vi "Reset Error Status.vi"(8 "error in (no error)":errorcluster, 11 "navX Error Status in":refnum<class "navX Error Status.lvclass">) -> (0 "error out":errorcluster, 3 "navX Error Status out":refnum<class "navX Error Status.lvclass">)   [LabVIEW 2015, in "navX Library v3.lvlib" / "navX Error Status.lvclass"]
uses:
  navX Error Status.lvclass
  navX Error Status.lvclass/navX Error Status.ctl
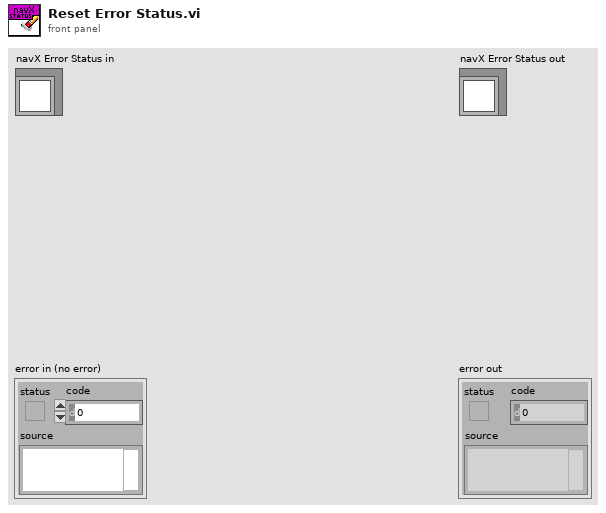
[diagram p1: front panel]
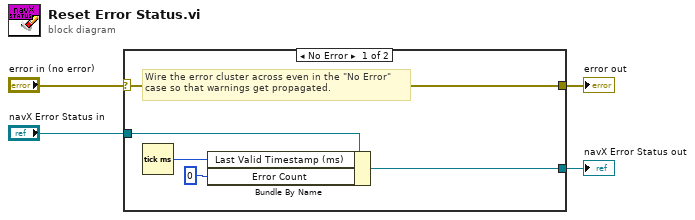
[diagram p0: block diagram]
diagram:
  n1 = case shown="No Error" "error in (no error)" {
    selector: "error in (no error)" -> [w8 w11]
    tunnel: [w8 w11] -> w3
    tunnel: [w7 w10] -> w1
    tunnel: "navX Error Status in" -> [w9 w10]
    frame No Error {
      # "Wire the error cluster across even in the \"No Error\"\ncase so that warnings get propagated."
      n2 = Tick Count (ms)() -> (millisecond timer value=w6:u32)
      n3 = Bundle By Name(cluster=w9, "Last Valid Timestamp (ms)"=w6, "Error Count"=0) -> (w7:refnum<class "navX Error Status.lvclass">)
    }
    frame Error {
    }
  }
  "error out" <- w3
  "navX Error Status out" <- w1
